vi "ProtectBall.vi"(0 "AlignSkill in":refnum<class "AlignSkill.lvclass">, 5 "Enemy":refnum<class "Robot.lvclass">, 7 "Robot":refnum<class "Robot.lvclass">, 9 "BallRef":refnum<class "Ball.lvclass">, 11 "error in (no error)":errorcluster, 12 "Skills.ProtectBall":cluster{"DistanceFromBall":dbl}) -> (4 "AlignSkill out":refnum<class "AlignSkill.lvclass">, 6 "Robot out":refnum<class "Robot.lvclass">, 15 "error out":errorcluster)   [LabVIEW 2023, in "AlignSkill.lvclass"]
uses:
  AlignSkill.lvclass
  Robot_class/Robot.lvclass
  C:/Users/ebert/Documents/codes/SSL/repo/SSL_AI/Object_class/Object.lvclass
  Ball_class/Ball.lvclass
  Object_class/Object.lvclass/Object.ctl
  <vilib>/Analysis/_algsub.llb/Real Vector Norm.vi
  Object_class/Read position(x,y).vi
  <vilib>/Analysis/NI_AALPro.lvlib
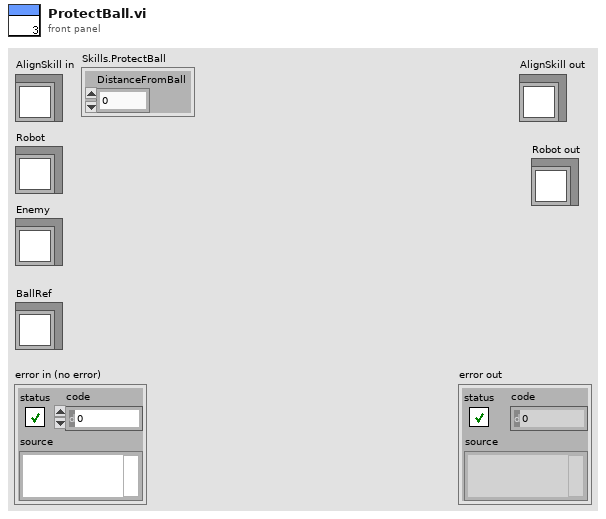
[diagram p1: front panel]
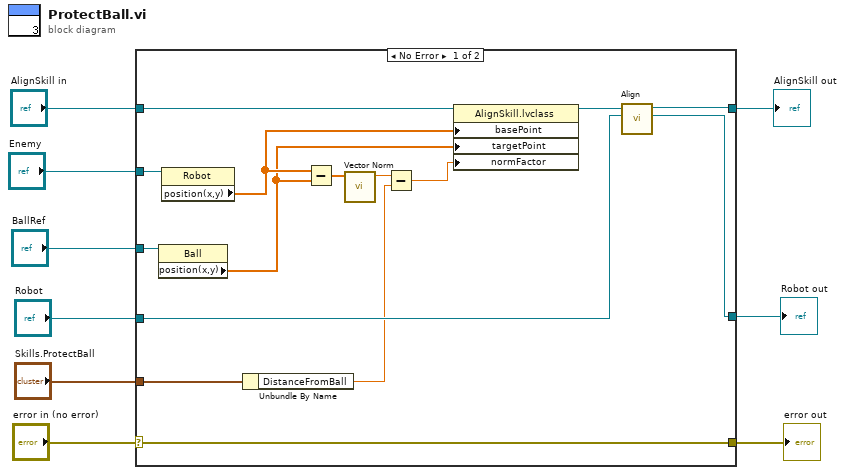
[diagram p0: block diagram]
diagram:
  n1 = case shown="No Error" "error in (no error)" {
    selector: "error in (no error)" -> [w24 w27]
    tunnel: [w24 w27] -> w8
    tunnel: [w23 w26] -> w6
    tunnel: "AlignSkill in" -> [w21 w26]
    tunnel: "Enemy" -> [w20 _]
    tunnel: "BallRef" -> [w19 _]
    tunnel: "Robot" -> [w13 w25]
    tunnel: [w12 w25] -> w2
    tunnel: "Skills.ProtectBall" -> [w11 _]
    frame No Error {
      n2 = property class="Ball"(reference=w19) -> ("position(x,y)"=w17:dbl[])  [unwired: 1 in, 2 out]
      n3 = property class="Robot"(reference=w20) -> ("position(x,y)"=w18:dbl[])  [unwired: 1 in, 2 out]
      n4 = Unbundle By Name(w11) -> ("DistanceFromBall"=w10:dbl)
      n5 = Subtract(x=w18, y=w17) -> (x-y=w16:dbl[])
      n6 = call-poly <vilib>:"Vector Norm.vi"("Input Vector"=w16) -> ("norm"=w15:dbl)  [unwired: 9 in, 1 out]
      n7 = Subtract(x=w15, y=w10) -> (x-y=w14:dbl)
      n8 = property class="AlignSkill.lvclass"(reference=w21, "basePoint"=w18, "targetPoint"=w17, "normFactor"=w14) -> (reference out=w22:refnum<class "AlignSkill.lvclass">)  [unwired: 1 in, 1 out]
      n9 = call-dynamic "Align.vi"("Robot"=w13, "AlignSkill in"=w22) -> ("Robot out"=w12:refnum<class "Robot.lvclass">, "AlignSkill out"=w23:refnum<class "AlignSkill.lvclass">)  [unwired: 7 in, 1 out]
    }
    frame Error {
    }
  }
  "error out" <- w8
  "AlignSkill out" <- w6
  "Robot out" <- w2
